vi "Wrong Count.vi"() -> (0 "error out":errorcluster)   [LabVIEW 2017, in "Assertion.Tests.lvlib" / "Assert Count.lvlib"]
uses:
  Assert Count.lvlib
  Assertion/Assertion.lvlib
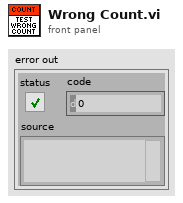
[diagram p1: front panel]
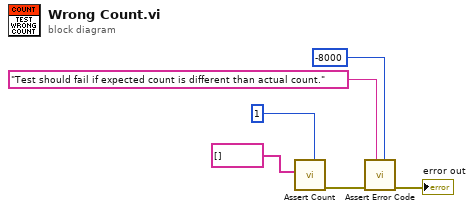
[diagram p0: block diagram]
diagram:
  n1 = call "Assert Count.vi"("Expected"=1, "Haystack"=string[] []) -> ("error out"=w1:errorcluster)  [unwired: 9 in]
  n2 = call "Assert Error Code.vi"("Expected"=-8000 ("code"), "Message (\"\")"="Test should fail if expected count is different than actual count." ("Message (\"\")"), "error in (no error)"=w1) -> ("error out"=→"error out":errorcluster)  [unwired: 8 in]
